vi "Get Sensor Units.vi"(8 "error in (no error)":errorcluster, 11 "Sensor List Class in":refnum<class "Sensor List Class.lvclass">) -> (0 "error out":errorcluster, 2 "Units":string[](array[string]), 3 "Sensor List Class out":refnum<class "Sensor List Class.lvclass">)   [LabVIEW 2013, in "Sensor List Class.lvclass"]
uses:
  Sensor List Class.lvclass
  Sensor DAO Class.lvclass/Sensor DAO Class.ctl
  Sensor DAO Class.lvclass
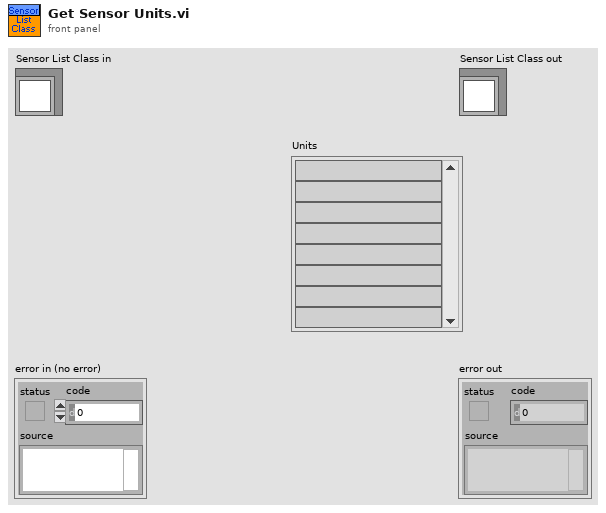
[diagram p1: front panel]
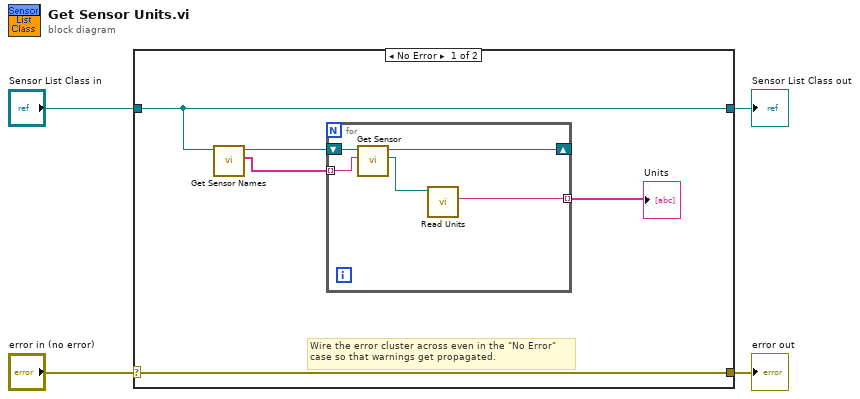
[diagram p0: block diagram]
diagram:
  n1 = case shown="No Error" "error in (no error)" {
    selector: "error in (no error)" -> [w9 w16]
    tunnel: [w9 w16] -> w3
    tunnel: [w8 w15] -> w1
    tunnel: "Sensor List Class in" -> [w8 w15]
    frame No Error {
      # "Wire the error cluster across even in the \"No Error\"\ncase so that warnings get propagated."
      n2 = call "Get Sensor Names.vi"("Sensor List Class in"=w8) -> ("Names"=w6:string[], "Sensor List Class out"=w7:refnum<class "Sensor List Class.lvclass">)  [unwired: 8 in, 1 out]
      n3 = for {
        shift-right: [w11] -> _
        shift-left: w7 -> [w14]
        tunnel: w6 -> [w13] mode=indexing
        tunnel: [w10] -> w5 mode=indexing
        n4 = call "Get Sensor.vi"("Name"=w13, "Sensor List Class in"=w14) -> ("Sensor DAO Out"=w12:refnum<class "Sensor DAO Class.lvclass">, "Sensor List Class out"=w11:refnum<class "Sensor List Class.lvclass">)  [unwired: 7 in, 1 out]
        n5 = call "Read Units.vi"("Sensor DAO Class in"=w12) -> ("Units"=w10:string)  [unwired: 8 in, 2 out]
      }
      "Units" <- w5
    }
    frame Error {
    }
  }
  "error out" <- w3
  "Sensor List Class out" <- w1
